vi "SubtractCrossCal.vi"(0 "slope (m)":dbl[][](array[numeric]) format="%.2f", 1 "intercept (b) out":dbl[][](array[numeric]) format="%.2f", 2 "midband fit in":dbl[][](array[numeric]) format="%.2f", 3 "Fit band":T1 {"center freq" format="%.2f"; "stop freq" format="%.2f"; "start" format="%.2f"}, 4 "Cross Cal":sgl[][](array[numeric]) format="%.2f") -> (5 "slope out":dbl[][](array[numeric]) format="%.2f", 6 "intercept out":dbl[][](array[numeric]) format="%.2f", 7 "midband fitout":dbl[][](array[numeric]) format="%.2f")   [LabVIEW 2022 SP3]
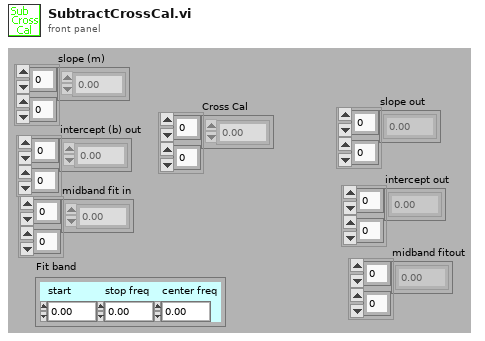
[diagram p1: front panel]
types:
  T1 = cluster{"start":dbl, "stop freq":dbl, "center freq":dbl}
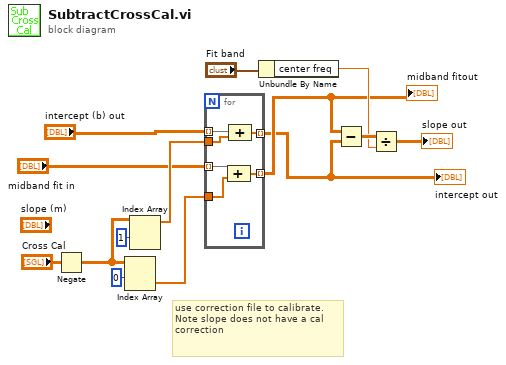
[diagram p0: block diagram]
diagram:
  # "use correction file to calibrate. Note slope does not have a cal correction"
  n1 = Negate(x="Cross Cal") -> (-x=w5:sgl[][])
  n2 = Index Array(array=w5, index (row)=0) -> (element=w10:sgl[])  [unwired: 1 in]
  n3 = Index Array(array=w5, index (row)=1) -> (element=w12:sgl[])  [unwired: 1 in]
  n4 = for {
    tunnel: "midband fit in" -> [w20] mode=indexing
    tunnel: [w19] -> w2 mode=indexing
    tunnel: w10 -> [w18]
    tunnel: w12 -> [w15]
    tunnel: "intercept (b) out" -> [w17] mode=indexing
    tunnel: [w16] -> w1 mode=indexing
    n5 = Compound Arithmetic op=unknown(w20, w18) -> (w19:dbl[])
    n6 = Compound Arithmetic op=unknown(w17, w15) -> (w16:dbl[])
  }
  "intercept out" <- w1
  "midband fitout" <- w2
  n7 = Unbundle By Name("Fit band") -> ("center freq"=w8:dbl)
  n8 = Subtract(x=w2, y=w1) -> (x-y=w9:dbl[][])
  n9 = Divide(x=w9, y=w8) -> (x/y=→"slope out":dbl[][])
